vi "Write_ini_file.vi"(2 "Section":string, 3 "error in (no error)":errorcluster, 4 "Element":string[](array[string]), 5 "Key":string[](array[string]), 6 "configuration file path":path) -> (0 "error out":errorcluster, 1 "found?":bool)   [LabVIEW 2022 SP3]
uses:
  <vilib>/Utility/config.llb/Write Key (String).vi
  <vilib>/Utility/config.llb/NI_LVConfig.lvlib
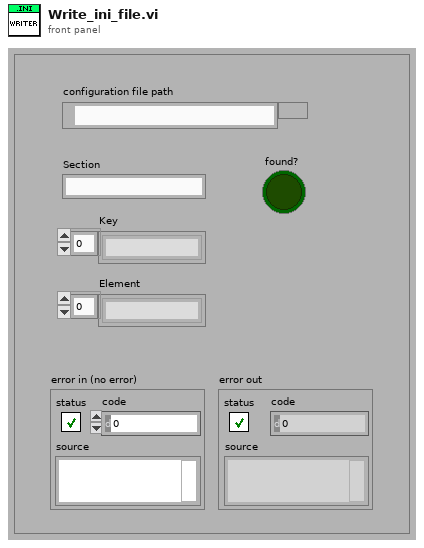
[diagram p1: front panel]
types:
  T1 = typedef "NI_LVConfig.lvlib/Config Data RefNum.ctl" = refnum<k1>
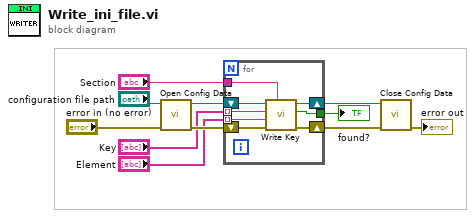
[diagram p0: block diagram]
diagram:
  n1 = call <vilib>:"Open Config Data.vi"("error in (no error)"="error in (no error)", "configuration file path"="configuration file path") -> ("error out"=w11:errorcluster, "refnum"=w9:T1)  [unwired: 7 in, 1 out]
  n2 = for {
    shift-right: [w16] -> w7
    shift-left: w11 -> [w19]
    shift-right: [w17] -> w8
    shift-left: w9 -> [w18]
    tunnel: [w15] -> w6
    tunnel: "Section" -> [w14]
    tunnel: "Key" -> [w13] mode=indexing
    tunnel: "Element" -> [w12] mode=indexing
    n3 = call-poly <vilib>:"Write Key.vi"("section"=w14, "error in (no error)"=w19, "value"=w12, "key"=w13, "refnum"=w18) -> ("error out"=w16:errorcluster, "found?"=w15:bool, "refnum out"=w17:T1)  [unwired: 4 in]
  }
  "found?" <- w6
  n4 = call <vilib>:"Close Config Data.vi"("error in (no error)"=w7, "refnum"=w8) -> ("error out"=→"error out":errorcluster)  [unwired: 8 in, 1 out]
